vi "Set IPS Fill Mode.vi"(8 "error in (no error)":errorcluster, 10 "Fill Mode":T1="ON", 11 "Instrument.Oxford1820 in":refnum<class "Instrument.Oxford1820.lvclass">) -> (0 "error out":errorcluster, 2 "Response":string, 3 "Instrument.Oxford1820 out":refnum<class "Instrument.Oxford1820.lvclass">)   [LabVIEW 2019, in "Instrument.Oxford1820.lvclass"]
uses:
  Instrument.Oxford1820.lvclass
  <instrlib>/Mercury iXX/Mercury iXX.lvlib
  <instrlib>/Mercury iXX/Public/Libraries/Level Meter/Configuration/Set/Pulse Slow-Fast (Set).vi
  <instrlib>/Mercury iXX/Public/Libraries/Level Meter.lvlib
  <instrlib>/Mercury iXX/Public/Libraries/Level Meter/Open/Open Level Meter Device.vi
  Typedefs/Fill Mode-Combo.ctl
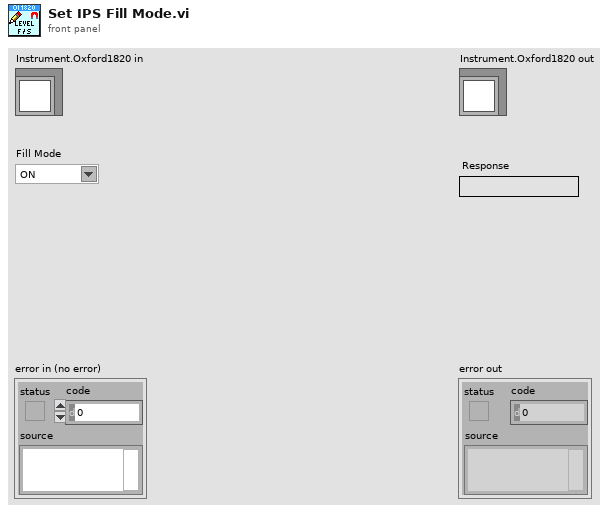
[diagram p1: front panel]
types:
  T1 = typedef "Instrument.Oxford1820.lvclass/Fill Mode-Combo.ctl" = string
  T2 = typedef "Mercury iXX.lvlib/Mercury Reference.ctl" = cluster{"Comms":refnum<visa-resource-name>, "Device ID":string[], "Comms Layer":T3, "Command":string, "Query reference":T4}
  T3 = typedef "Mercury iXX.lvlib/Comms Transport Layer.ctl" = enum16{"Ethernet TCP/IP", "USB", "ISOBus - RS-232", "GPIB"}
  T4 = typedef "Mercury iXX.lvlib/Query Dynamic Reference.ctl" = refnum<vi>
  T5 = typedef "Mercury iXX.lvlib/Response String.ctl" = string
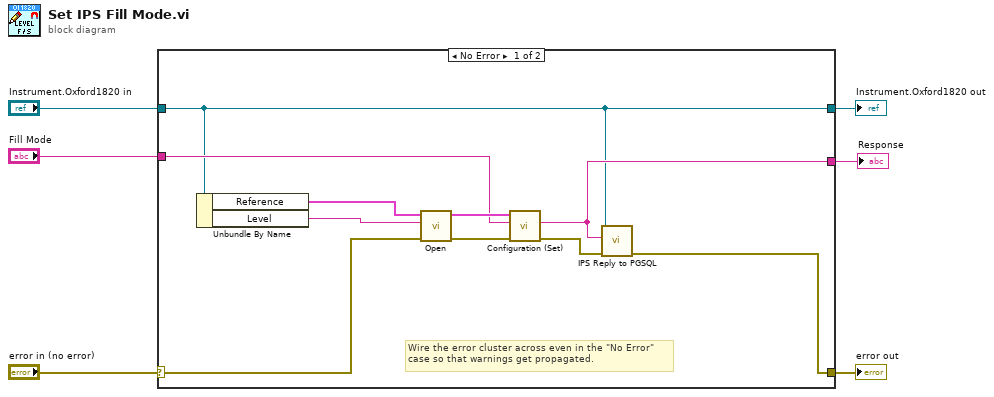
[diagram p0: block diagram]
diagram:
  n1 = case shown="No Error" "error in (no error)" {
    selector: "error in (no error)" -> [w10 w18]
    tunnel: [w8 w18] -> w5
    tunnel: [w7 w17] -> w3
    tunnel: "Instrument.Oxford1820 in" -> [w7 w17]
    tunnel: [w9 _] -> w2
    tunnel: "Fill Mode" -> [w13 _]
    frame No Error {
      # "Wire the error cluster across even in the \"No Error\"\ncase so that warnings get propagated."
      n2 = Unbundle By Name(w7) -> ("Reference"=w12:T2, "Level"=w11:string)
      n3 = call-poly <instrlib>:"Open.vi"("error in (no error)"=w10, "Device Identifier"=w11, "Mercury Reference In"=w12) -> ("error out"=w15:errorcluster, "Mercury Reference Out"=w14:T2)  [unwired: 7 out]
      n4 = call-poly <instrlib>:"Configuration (Set).vi"("error in"=w15, "Delay"=w13, "Mercury Reference In"=w14) -> ("error out"=w16:errorcluster, "Response"=w9:T5)  [unwired: 5 in, 2 out]
      n5 = call "IPS Reply to PGSQL.vi"("error in (no error)"=w16, "Response"=w9, "Instrument.1820 in"=w7) -> ("error out"=w8:errorcluster)  [unwired: 7 in, 1 out]
    }
    frame Error {
    }
  }
  "error out" <- w5
  "Instrument.Oxford1820 out" <- w3
  "Response" <- w2
